vi "LNLS Control Decode FOFBC.vi"(8 "error in (no error)":errorcluster, 10 "command body":string) -> (0 "error out":errorcluster, 3 "LNLS Control FOFB Configuration":T1)   [LabVIEW 2011, in "LNLS Control VIs.lvlib"]
uses:
  LNLS Control VIs.lvlib
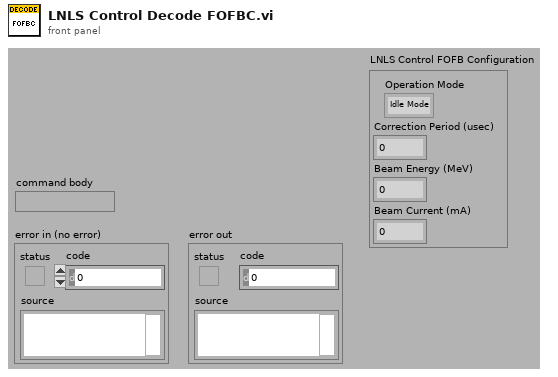
[diagram p1: front panel]
types:
  T1 = cluster{"Operation Mode":enum16{"Idle Mode", "Error Mode", "Manual Mode", "FOFB Mode", "RMM Mode"}, "Correction Period (usec)":i32, "Beam Energy (MeV)":sgl, "Beam Current (mA)":sgl}
  T2 = enum16{"Idle Mode", "Error Mode", "Manual Mode", "FOFB Mode", "RMM Mode"}
  T3 = enum16{"big-endian, network order", "native, host order", "little-endian"}
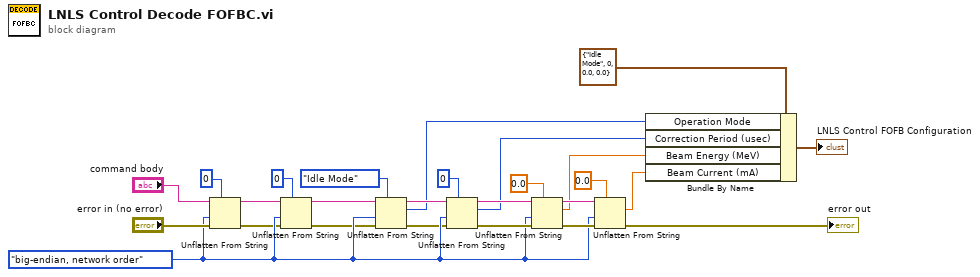
[diagram p0: block diagram]
diagram:
  w21 = T3."big-endian, network order" ("byte order (0:big-endian, network order)")
  n1 = Unflatten From String(type=u8 0 ("priority"), binary string="command body", byte order (0:big-endian, network order)=w21, error in (no error)="error in (no error)") -> (rest of the binary string=w17:string, error out=w16:errorcluster)  [unwired: 1 in, 1 out]
  n2 = Unflatten From String(type=u8 0 ("flag"), binary string=w17, byte order (0:big-endian, network order)=w21, error in (no error)=w16) -> (rest of the binary string=w9:string, error out=w10:errorcluster)  [unwired: 1 in, 1 out]
  n3 = Unflatten From String(type=T2."Idle Mode" ("Current Operation Mode"), binary string=w9, byte order (0:big-endian, network order)=w21, error in (no error)=w10) -> (rest of the binary string=w6:string, value=w1:T2, error out=w8:errorcluster)  [unwired: 1 in]
  n4 = Unflatten From String(type=0 ("Correction Period (usec)"), binary string=w6, byte order (0:big-endian, network order)=w21, error in (no error)=w8) -> (rest of the binary string=w7:string, value=w2:i32, error out=→"error out":errorcluster)  [unwired: 1 in]
  n5 = Unflatten From String(type=sgl 0.0 ("Beam Energy (MeV)"), binary string=w7, byte order (0:big-endian, network order)=w21) -> (rest of the binary string=w11:string, value=w4:sgl)  [unwired: 2 in, 1 out]
  n6 = Unflatten From String(type=sgl 0.0 ("Beam Current (mA)"), binary string=w11, byte order (0:big-endian, network order)=w21) -> (value=w3:sgl)  [unwired: 2 in, 2 out]
  n7 = Bundle By Name(cluster=T1 {"Operation Mode"=enum."Idle Mode", "Correction Period (usec)"=0, "Beam Energy (MeV)"=0.0, "Beam Current (mA)"=0.0} ("LNLS Control FOFB Configuration 2"), "Operation Mode"=w1, "Correction Period (usec)"=w2, "Beam Energy (MeV)"=w4, "Beam Current (mA)"=w3) -> (→"LNLS Control FOFB Configuration":T1)
